vi "test_memory_leak_parr_VI.vi"() -> ()   [LabVIEW 2020]
panel:
  out "# VI in work":i32
  in  "how long is array":i32=100
  in  "# VIs":i32=10
  in  "VI in parrallel":bool
  out "Iter data generation":i32
  in  "Clean":bool
  in  "Add":bool
  in  "stop":bool
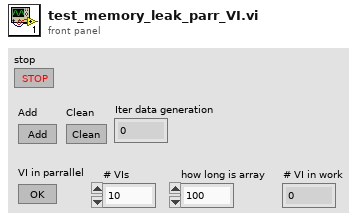
[diagram p1: front panel]
types:
  T1 = cluster{"Data Raw":dbl[][][][], "data value reference":refnum<data-value>}
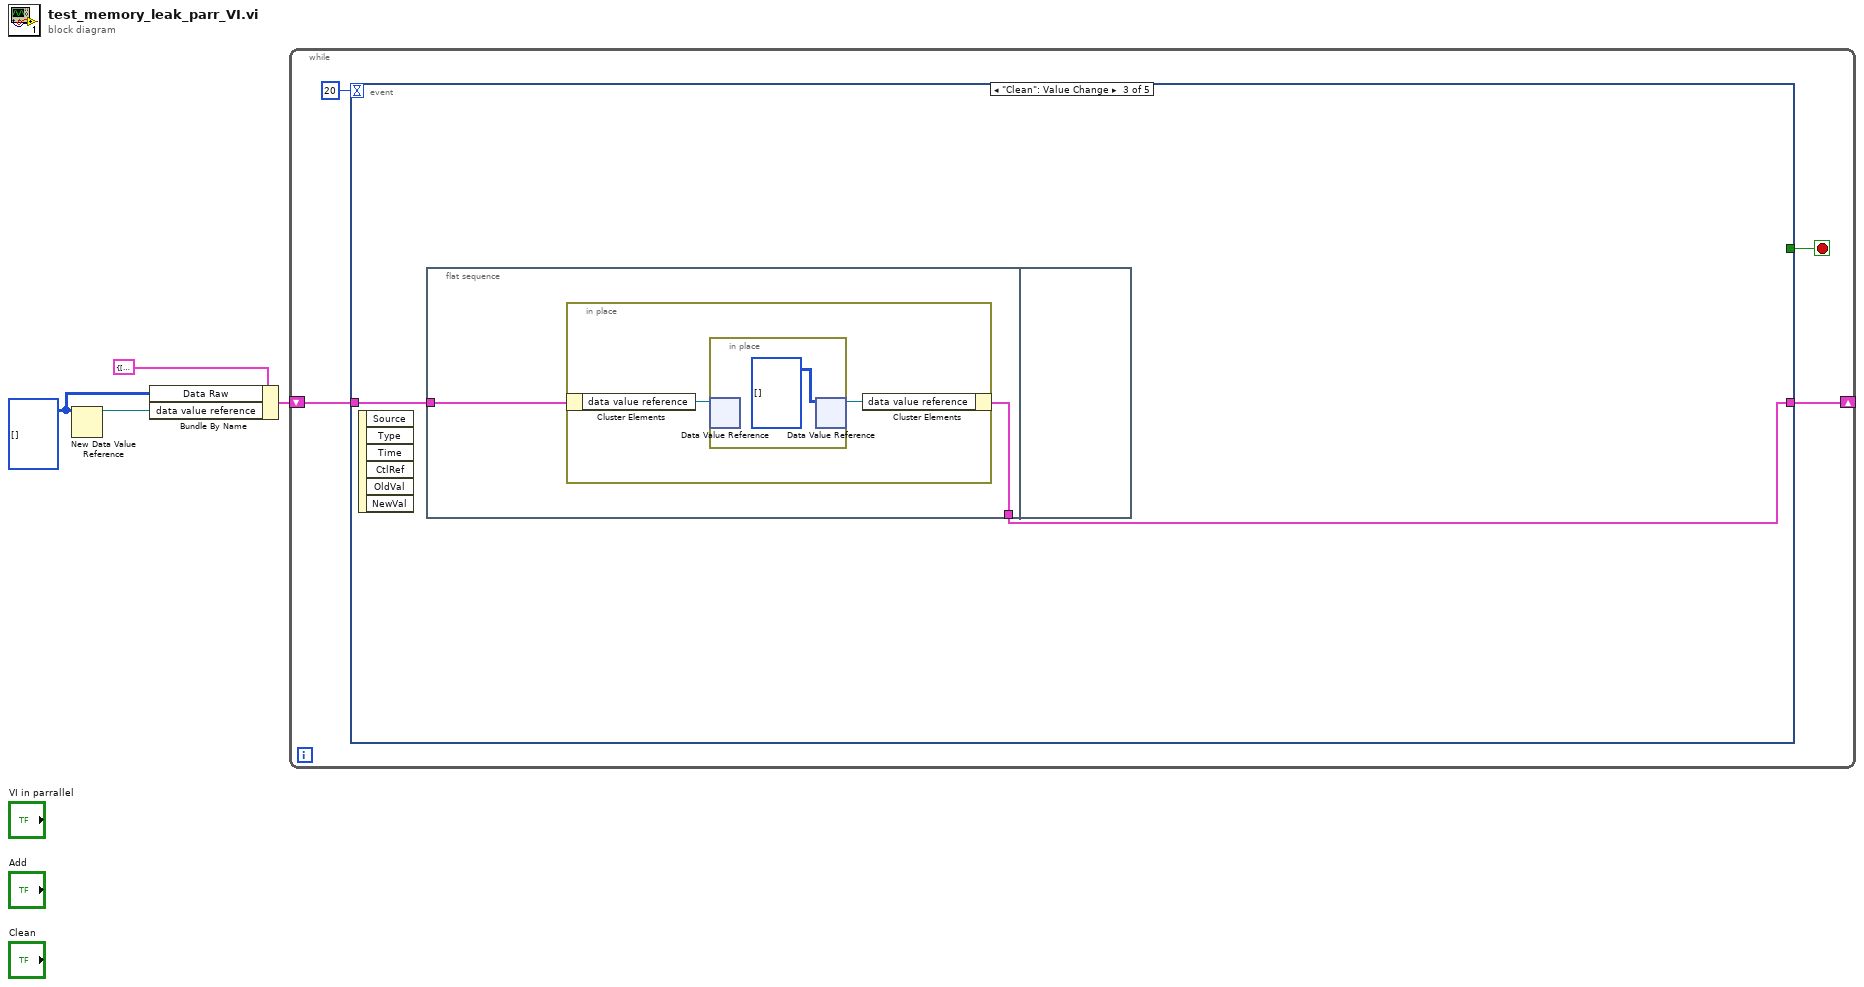
[diagram p0: block diagram]
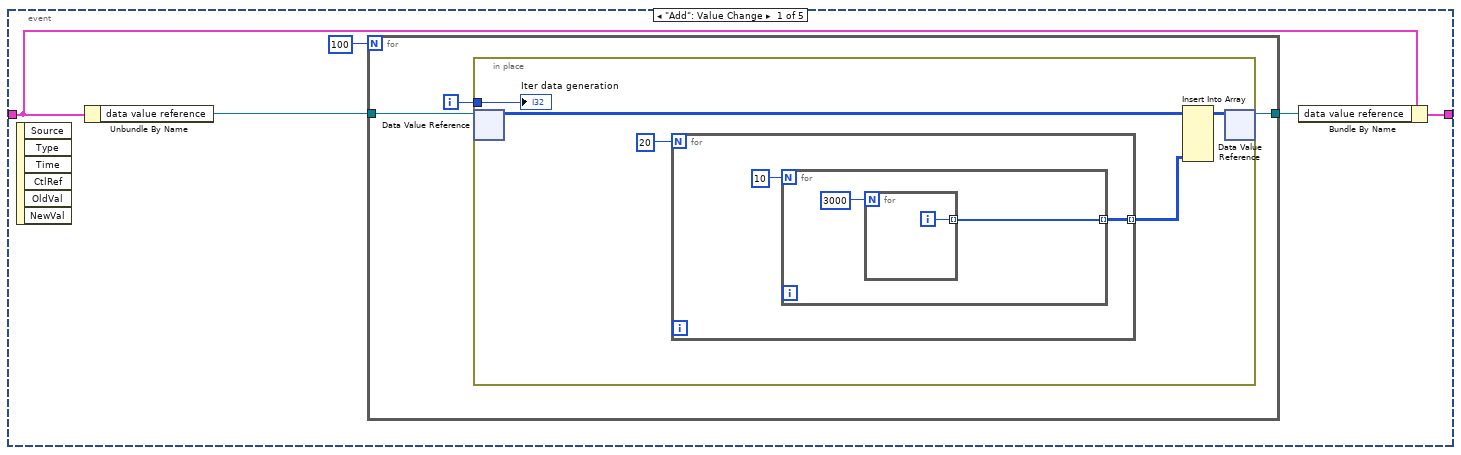
[diagram p2: hidden frame]
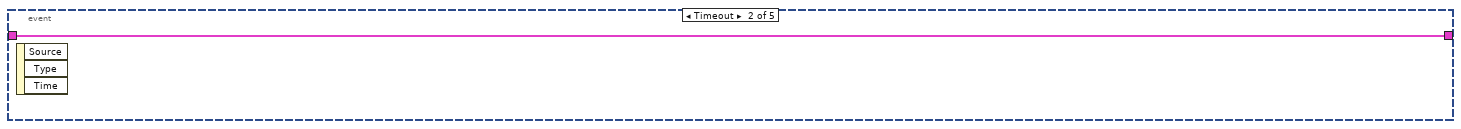
[diagram p3: hidden frame]
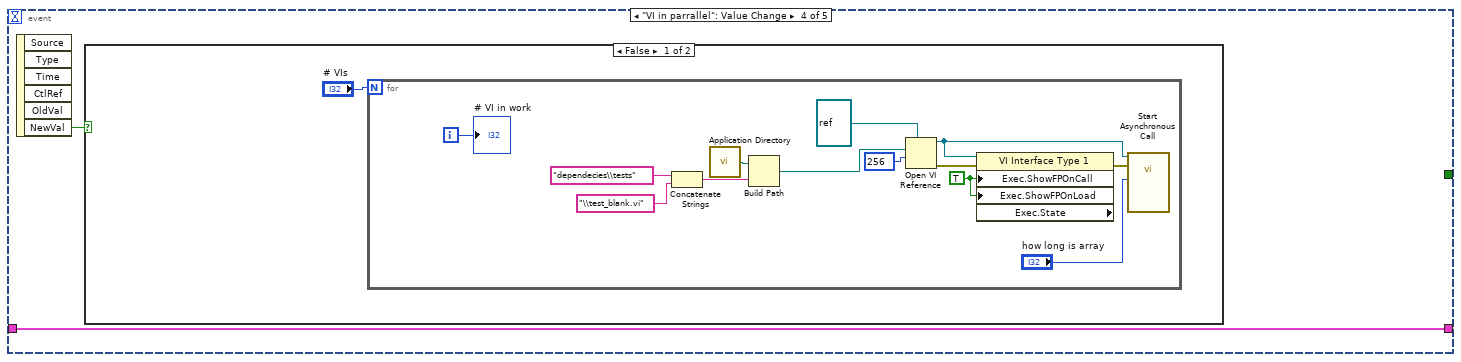
[diagram p4: hidden frame]
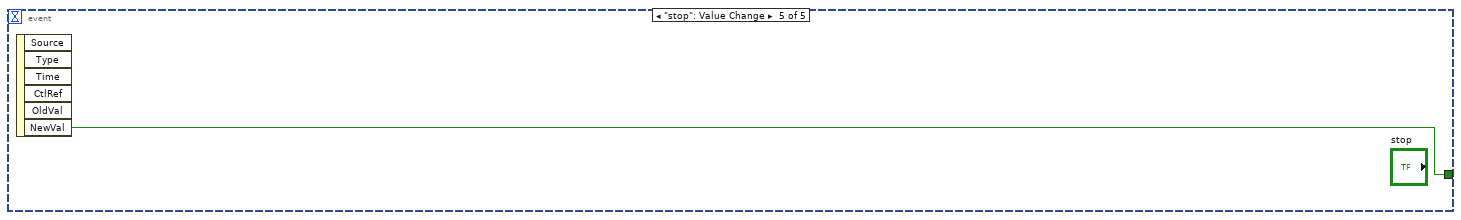
[diagram p6: hidden frame]
diagram:
  w2 = i32[][][][] [] ("Data Raw")
  n1 = New Data Value Reference(data value=w2) -> (data value reference=w1:refnum<data-value>)  [unwired: 1 in, 1 out]
  n2 = Bundle By Name(cluster=T1 {"Data Raw"=[], "data value reference"=refnum}, "Data Raw"=w2, "data value reference"=w1) -> (w3:T1)
  n3 = while {
    shift-right: [w7] -> _
    shift-left: w3 -> [w6]
    stop <- w5 stop-if-true
    n4 = event shown="[2] \"Clean\": Value Change" {
      selector: _ -> [_ _ _ _ _]
      dyn-events: _ -> [_ _ _ _ _]
      timeout: 20 -> [_ _ _ _ _]
      tunnel: [w12 w27 w28 w35 _] -> w7
      tunnel: w6 -> [w11 w27 w29 w35 _]
      tunnel: [_ _ _ _ w51] -> w5
      event "Add": Value Change {
        n5 = event-data() -> ()  [unwired: 1 in, 6 out]
        n6 = Unbundle By Name(w11) -> ("data value reference"=w10:refnum<data-value>)
        n7 = for {
          N: 100 -> [_]
          tunnel: w10 -> [w15]
          tunnel: [w14] -> w9
          i -> [w16]
          n8 = in-place {
            in-place-border: w16 -> [w20]
            n9 = in-place-dvr #1(w15) -> (w18:i32[][][][])  [unwired: 1 out]
            n10 = for {
              N: 20 -> [_]
              tunnel: [w23] -> w19 mode=indexing
              n11 = for {
                N: 10 -> [_]
                tunnel: [w25] -> w23 mode=indexing
                n12 = for {
                  N: 3000 -> [_]
                  tunnel: [w26] -> w25 mode=indexing
                  i -> [w26]
                }
              }
            }
            n13 = Insert Into Array(array=w18, new element=w19) -> (w17:i32[][][][])  [unwired: 4 in]
            n14 = in-place-dvr #1(w17) -> (w14:refnum<data-value>)  [unwired: 1 out]
            "Iter data generation" <- w20
          }
        }
        n15 = Bundle By Name(cluster=w11, "data value reference"=w9) -> (w12:T1)
      }
      event Timeout {
        n16 = event-data() -> ()  [unwired: 1 in, 3 out]
      }
      event "Clean": Value Change {
        n17 = event-data() -> ()  [unwired: 1 in, 6 out]
        n18 = flat-sequence {
          tunnel: w29 -> [w31]
          tunnel: [w30] -> w28
          frame #0 {
            n19 = in-place {
              n20 = in-place-cluster #2(w31) -> ("data value reference"=w33:refnum<data-value>)
              n21 = in-place {
                n22 = in-place-dvr #3(w33) -> ()  [unwired: 2 out]
                n23 = in-place-dvr #3(i32[][][][] [] ("data value")) -> (w32:refnum<data-value>)  [unwired: 1 out]
              }
              n24 = in-place-cluster #2("data value reference"=w32) -> (w30:T1)
            }
          }
          frame #1 {
          }
        }
      }
      event "VI in parrallel": Value Change {
        n25 = event-data() -> ("NewVal"=w36:bool)  [unwired: 1 in, 5 out]
        n26 = case shown="False" w36 {
          frame False {
            n27 = for {
              N: "# VIs" -> [_]
              i -> [w38]
              w48 = TRUE ("Execution:Show Front Panel On Call")
              n28 = Concatenate Strings("dependecies\\tests" ("chaîne"), "\\test_blank.vi" ("chaîne")) -> (w44:string)
              n29 = call <vilib>:"Application Directory.vi"() -> ("Application Directory"=w45:path)
              n30 = Build Path(base path=w45, name or relative path=w44) -> (appended path=w41:path)
              n31 = Open VI Reference(type specifier VI Refnum (for type only)=refnum<vi> refnum ("spécificateur de type du refnum de VI (pour type seulement)"), vi path=w41, options=256) -> (vi reference=w49:refnum<vi>, error out=w47:errorcluster)  [unwired: 3 in]
              n32 = property class="VI Interface Type 1" props=["Exec.ShowFPOnCall", "Exec.ShowFPOnLoad", "Exec.State"](reference=w49, error in=w47, "Exec.ShowFPOnCall"=w48, "Exec.ShowFPOnLoad"=w48) -> (error out=w39:errorcluster)  [unwired: 2 out]
              n33 = call-by-ref "Start Asynchronous Call"(reference=w49, error in=w39, "number"="how long is array") -> ()  [unwired: 11 in, 2 out]
              "# VI in work" <- w38
            }
          }
          frame True {
          }
        }
      }
      event "stop": Value Change {
        n34 = event-data() -> ("NewVal"=w51:bool)  [unwired: 1 in, 5 out]
      }
    }
  }
